vi "move.vi"(8 "error in (no error)":errorcluster, 9 "y":i32, 10 "x":i32, 11 "Circle in":refnum<class "Circle.lvclass">) -> (0 "error out":errorcluster, 3 "Circle out":refnum<class "Circle.lvclass">)   [LabVIEW 2017, in "Circle.lvclass"]
uses:
  Circle.lvclass
  Shape Class/Shape.lvclass
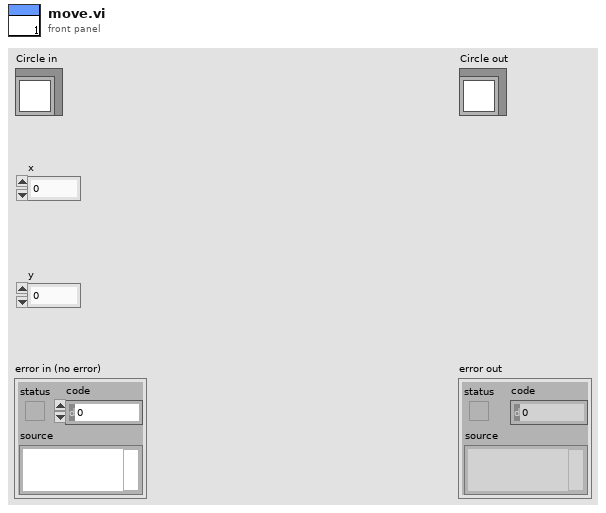
[diagram p1: front panel]
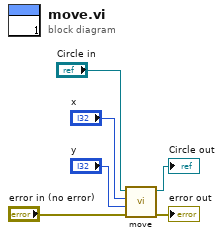
[diagram p0: block diagram]
diagram:
  n1 = call-parent "move.vi"("error in (no error)"="error in (no error)", "y"="y", "x"="x", "Shape in"="Circle in") -> ("error out"=→"error out":errorcluster, "Shape out"=→"Circle out":refnum<class "Circle.lvclass">)  [unwired: 6 in]
